vi "Dialog.Name.CheckErrors.vi"(7 "Existing Frames":string[](array[string]), 8 "error in (no error)":errorcluster, 10 "ID":u16, 11 "Name":string) -> (0 "error out":errorcluster, 2 "Error":string, 3 "Error?":bool)   [LabVIEW 2019, in "Diagnostics Addon System Explorer.lvlib"]
uses:
  Diagnostics Addon System Explorer.lvlib
  Frame.Convert.Name.vi
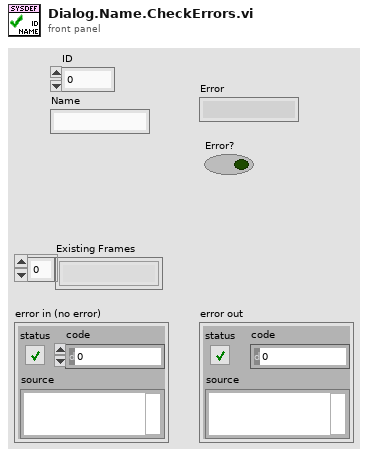
[diagram p1: front panel]
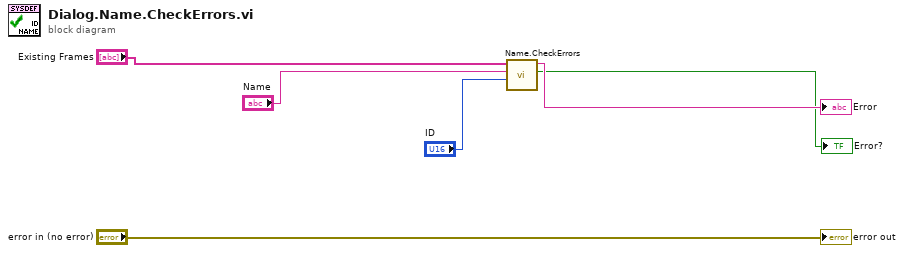
[diagram p0: block diagram]
diagram:
  n1 = call "Name.CheckErrors.vi"("ID"="ID", "Name"="Name", "Existing Frames"="Existing Frames") -> ("Error?"=→"Error?":bool, "Error String"=→"Error":string)  [unwired: 7 in]
  "error out" <- "error in (no error)"
